vi "Load INI Config.vi"(8 "error in":errorcluster, 11 "configuration file path":path) -> (0 "error out":errorcluster)   [LabVIEW 2021]
uses:
  Controls/MUX_Data.ctl
  Controls/Keysight6700C_Data.ctl
  Controls/DMM_Data.ctl
  Controls/DAQ_Data.ctl
  Controls/Instruments Cluster.ctl
  <vilib>/Utility/config.llb/Read Key (String).vi
  <vilib>/Utility/config.llb/NI_LVConfig.lvlib
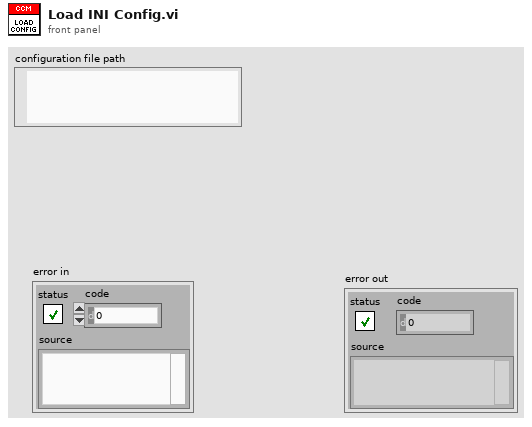
[diagram p1: front panel]
types:
  T1 = typedef "NI_LVConfig.lvlib/Config Data RefNum.ctl" = refnum<k1>
  T2 = typedef "MUX_Data.ctl" = cluster{"Alias":string, "Topology":string}
  T3 = typedef "Keysight6700C_Data.ctl" = cluster{"Alias":string, "Device":string, "Channel name":string}
  T4 = typedef "DMM_Data.ctl" = cluster{"Alias":string, "MUX":string, "Route":string}
  T5 = typedef "DAQ_Data.ctl" = cluster{"Alias":string, "DAQ Ch":string}
  T6 = typedef "Instruments Cluster.ctl" = cluster{"Alias":string, "Address/SN":string, "Channel":string}
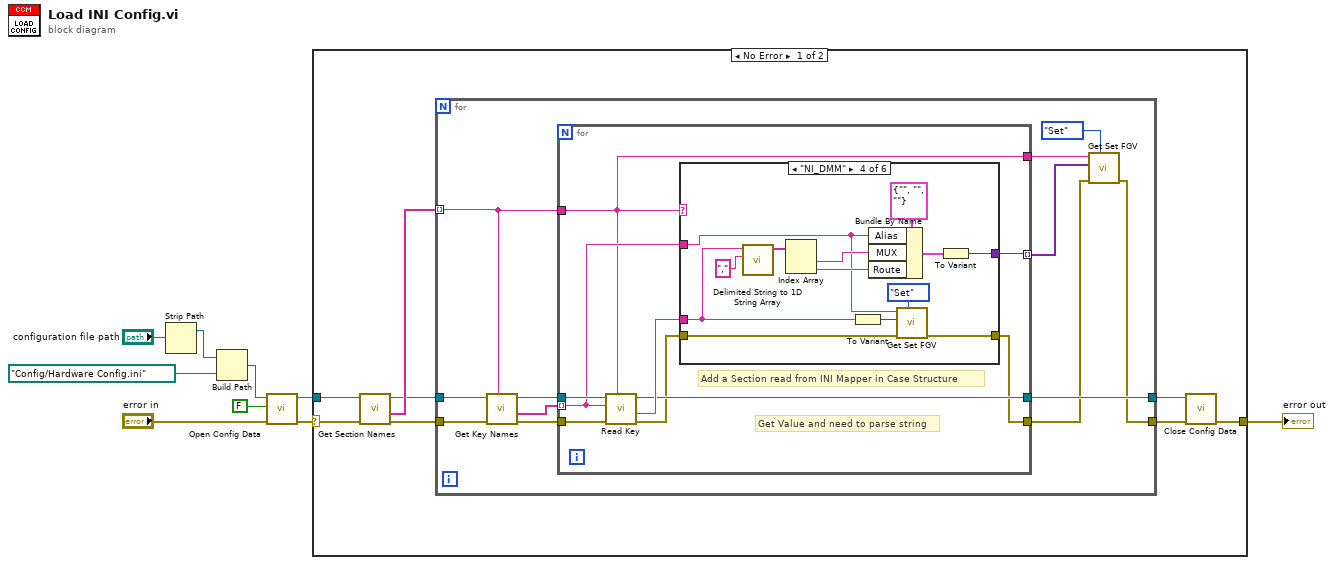
[diagram p0: block diagram]
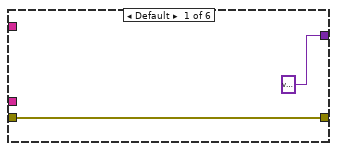
[diagram p2: hidden frame]
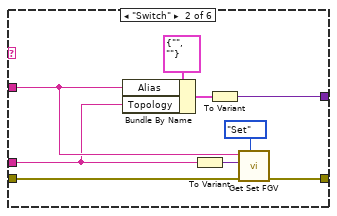
[diagram p3: hidden frame]
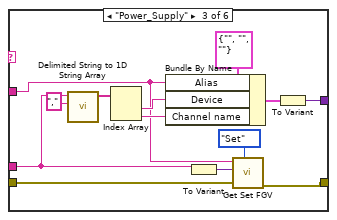
[diagram p4: hidden frame]
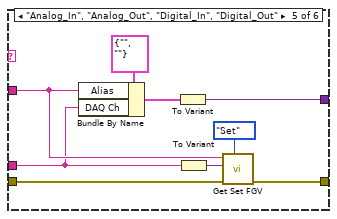
[diagram p5: hidden frame]
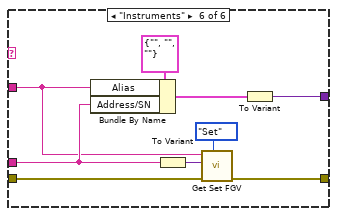
[diagram p6: hidden frame]
diagram:
  n1 = Strip Path(path="configuration file path") -> (stripped path=w2:path)  [unwired: 1 out]
  n2 = Build Path(base path=w2, name or relative path=path "Config/Hardware Config.ini") -> (appended path=w4:path)
  n3 = call <vilib>:"Open Config Data.vi"("error in (no error)"="error in", "create file if necessary (T)"=FALSE, "configuration file path"=w4) -> ("error out"=w7:errorcluster, "refnum"=w8:T1)  [unwired: 6 in, 1 out]
  n4 = case shown="No Error" w7 {
    selector: w7 -> [w17 w94]
    tunnel: [w10 w94] -> w1
    tunnel: w8 -> [w16 _]
    frame No Error {
      n5 = call <vilib>:"Get Section Names.vi"("error in (no error)"=w17, "refnum"=w16) -> ("error out"=w14:errorcluster, "section names"=w15:string[], "refnum out"=w13:T1)  [unwired: 7 in]
      n6 = for {
        tunnel: w15 -> [w26] mode=indexing
        tunnel: w14 -> [w29]
        tunnel: w13 -> [w28]
        tunnel: [w27] -> w12
        tunnel: [w19] -> w11
        n7 = call <vilib>:"Get Key Names.vi"("section"=w26, "error in (no error)"=w29, "refnum"=w28) -> ("error out"=w25:errorcluster, "key names"=w24:string[], "refnum out"=w23:T1)  [unwired: 5 in, 1 out]
        n8 = for {
          tunnel: w24 -> [w36] mode=indexing
          tunnel: w26 -> [w32]
          tunnel: w23 -> [w37]
          tunnel: [w34] -> w27
          tunnel: [w33] -> w21 mode=indexing
          tunnel: w25 -> [w38]
          tunnel: [w30] -> w20
          tunnel: [w32] -> w18
          # "Add a Section read from INI Mapper in Case Structure"
          # "Get Value and need to parse string"
          n9 = call-poly <vilib>:"Read Key.vi"("section"=w32, "error in (no error)"=w38, "key"=w36, "refnum"=w37) -> ("error out"=w31:errorcluster, "value"=w35:string, "refnum out"=w34:T1)  [unwired: 4 in, 1 out]
          n10 = case shown="\"NI_DMM\"" w32 {
            tunnel: w36 -> [_ w43 w50 w63 w79 w85]
            tunnel: w35 -> [_ w42 w51 w64 w78 w88]
            tunnel: [variant ("Variant") w48 w62 w71 w84 w86] -> w33
            tunnel: w31 -> [w39 w41 w53 w65 w77 w91]
            tunnel: [w39 w45 w52 w66 w76 w90] -> w30
            frame Default {
            }
            frame "Switch" {
              n11 = Bundle By Name(cluster=T2 {"Alias"="", "Topology"=""}, "Alias"=w43, "Topology"=w42) -> (w47:T2)
              n12 = To Variant(anything=w42) -> (Variant=w46:variant)
              n13 = To Variant(anything=w47) -> (Variant=w48:variant)
              n14 = call "Get Set FGV.vi"("Method (Get)"=enum16{"Get", "Set"}."Set", "error in"=w41, "Data In"=w46, "Name"=w43) -> ("error out"=w45:errorcluster)  [unwired: 6 in, 1 out]
            }
            frame "Power_Supply" {
              n15 = call <vilib>:"Delimited String to 1D String Array.vi"("delimiter"=",", "delimited string"=w51) -> ("string array"=w59:string[])  [unwired: 9 in]
              n16 = Index Array(array=w59) -> (element #1=w57:string, element #2=w56:string)  [unwired: 2 in]
              n17 = Bundle By Name(cluster=T3 {"Alias"="", "Device"="", "Channel name"=""} ("DAQ Data"), "Alias"=w50, "Device"=w57, "Channel name"=w56) -> (w60:T3)
              n18 = To Variant(anything=w51) -> (Variant=w55:variant)
              n19 = call "Get Set FGV.vi"("Method (Get)"=enum16{"Get", "Set"}."Set", "error in"=w53, "Data In"=w55, "Name"=w50) -> ("error out"=w52:errorcluster)  [unwired: 6 in, 1 out]
              n20 = To Variant(anything=w60) -> (Variant=w62:variant)
            }
            frame "NI_DMM" {
              n21 = call <vilib>:"Delimited String to 1D String Array.vi"("delimiter"=",", "delimited string"=w64) -> ("string array"=w74:string[])  [unwired: 9 in]
              n22 = Index Array(array=w74) -> (element #1=w70:string, element #2=w69:string)  [unwired: 2 in]
              n23 = To Variant(anything=w64) -> (Variant=w68:variant)
              n24 = Bundle By Name(cluster=T4 {"Alias"="", "MUX"="", "Route"=""} ("DAQ Data"), "Alias"=w63, "MUX"=w70, "Route"=w69) -> (w72:T4)
              n25 = call "Get Set FGV.vi"("Method (Get)"=enum16{"Get", "Set"}."Set", "error in"=w65, "Data In"=w68, "Name"=w63) -> ("error out"=w66:errorcluster)  [unwired: 6 in, 1 out]
              n26 = To Variant(anything=w72) -> (Variant=w71:variant)
            }
            frame "Analog_In", "Analog_Out", "Digital_In", "Digital_Out" {
              n27 = Bundle By Name(cluster=T5 {"Alias"="", "DAQ Ch"=""} ("DAQ Data"), "Alias"=w79, "DAQ Ch"=w78) -> (w82:T5)
              n28 = To Variant(anything=w82) -> (Variant=w84:variant)
              n29 = To Variant(anything=w78) -> (Variant=w81:variant)
              n30 = call "Get Set FGV.vi"("Method (Get)"=enum16{"Get", "Set"}."Set", "error in"=w77, "Data In"=w81, "Name"=w79) -> ("error out"=w76:errorcluster)  [unwired: 6 in, 1 out]
            }
            frame "Instruments" {
              n31 = Bundle By Name(cluster=T6 {"Alias"="", "Address/SN"="", "Channel"=""} ("Instruments Cluster"), "Alias"=w85, "Address/SN"=w88) -> (w87:T6)
              n32 = To Variant(anything=w88) -> (Variant=w92:variant)
              n33 = call "Get Set FGV.vi"("Method (Get)"=enum16{"Get", "Set"}."Set", "error in"=w91, "Data In"=w92, "Name"=w85) -> ("error out"=w90:errorcluster)  [unwired: 6 in, 1 out]
              n34 = To Variant(anything=w87) -> (Variant=w86:variant)
            }
          }
        }
        n35 = call "Get Set FGV.vi"("Method (Get)"=enum16{"Get", "Set"}."Set", "error in"=w20, "Data In"=w21, "Name"=w18) -> ("error out"=w19:errorcluster)  [unwired: 6 in, 1 out]
      }
      n36 = call <vilib>:"Close Config Data.vi"("error in (no error)"=w11, "refnum"=w12) -> ("error out"=w10:errorcluster)  [unwired: 8 in, 1 out]
    }
    frame Error {
    }
  }
  "error out" <- w1
